vi "StellarNet sw.ini Params.vi"(8 "Error State (In)":errorcluster, 11 "configuration file path":path=path "C:/program files/StellarNet/SpectraWiz/sw.ini") -> (0 "Error State (Out)":errorcluster, 1 "Channel Specific Data- Truncation Settings":cluster{"value":i32, "value":i32}[](array[cluster]), 2 "Channel\nParameters":T1(array[cluster]), 3 "Number of Channels":i32=3, 4 "Spectrometer Wavelengths":dbl[][](array[numeric]) format="%.2f", 5 "file or folder exists?":bool, 7 "Coefficients":ext[][](array[numeric]))   [LabVIEW 2023]
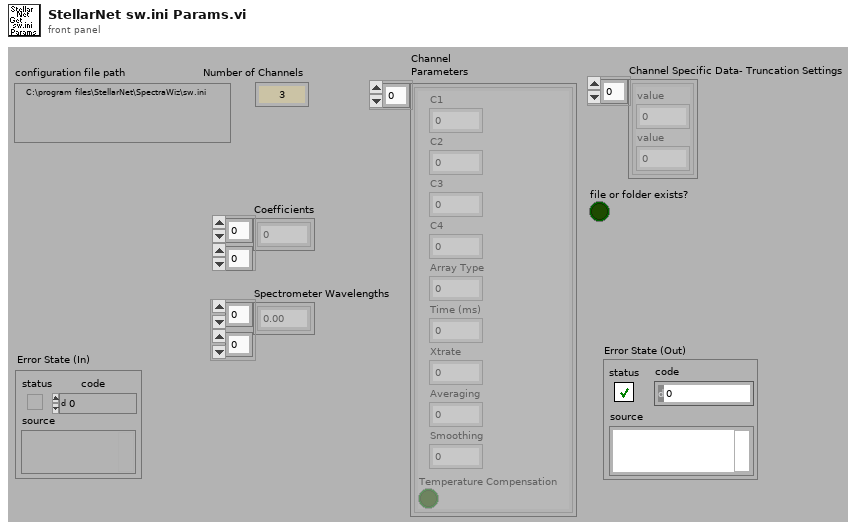
[diagram p1: front panel]
types:
  T1 = cluster{"C1":dbl, "C2":dbl, "C3":dbl, "C4":dbl, "Array Type":u16, "Time (ms)":i32, "Xtrate":i32, "Averaging":i32, "Smoothing":i32, "Temperature Compensation":bool}[]
  T2 = cluster{"C1":dbl, "C2":dbl, "C3":dbl, "C4":dbl, "Array Type":u16, "Time (ms)":i32, "Xtrate":i32, "Averaging":i32, "Smoothing":i32, "Temperature Compensation":bool}
  T3 = cluster{"[0]":dbl, "[1]":dbl, "[2]":dbl, "[3]":dbl, "[4]":dbl, "[5]":dbl, "[6]":dbl, "[7]":dbl, "[8]":dbl}
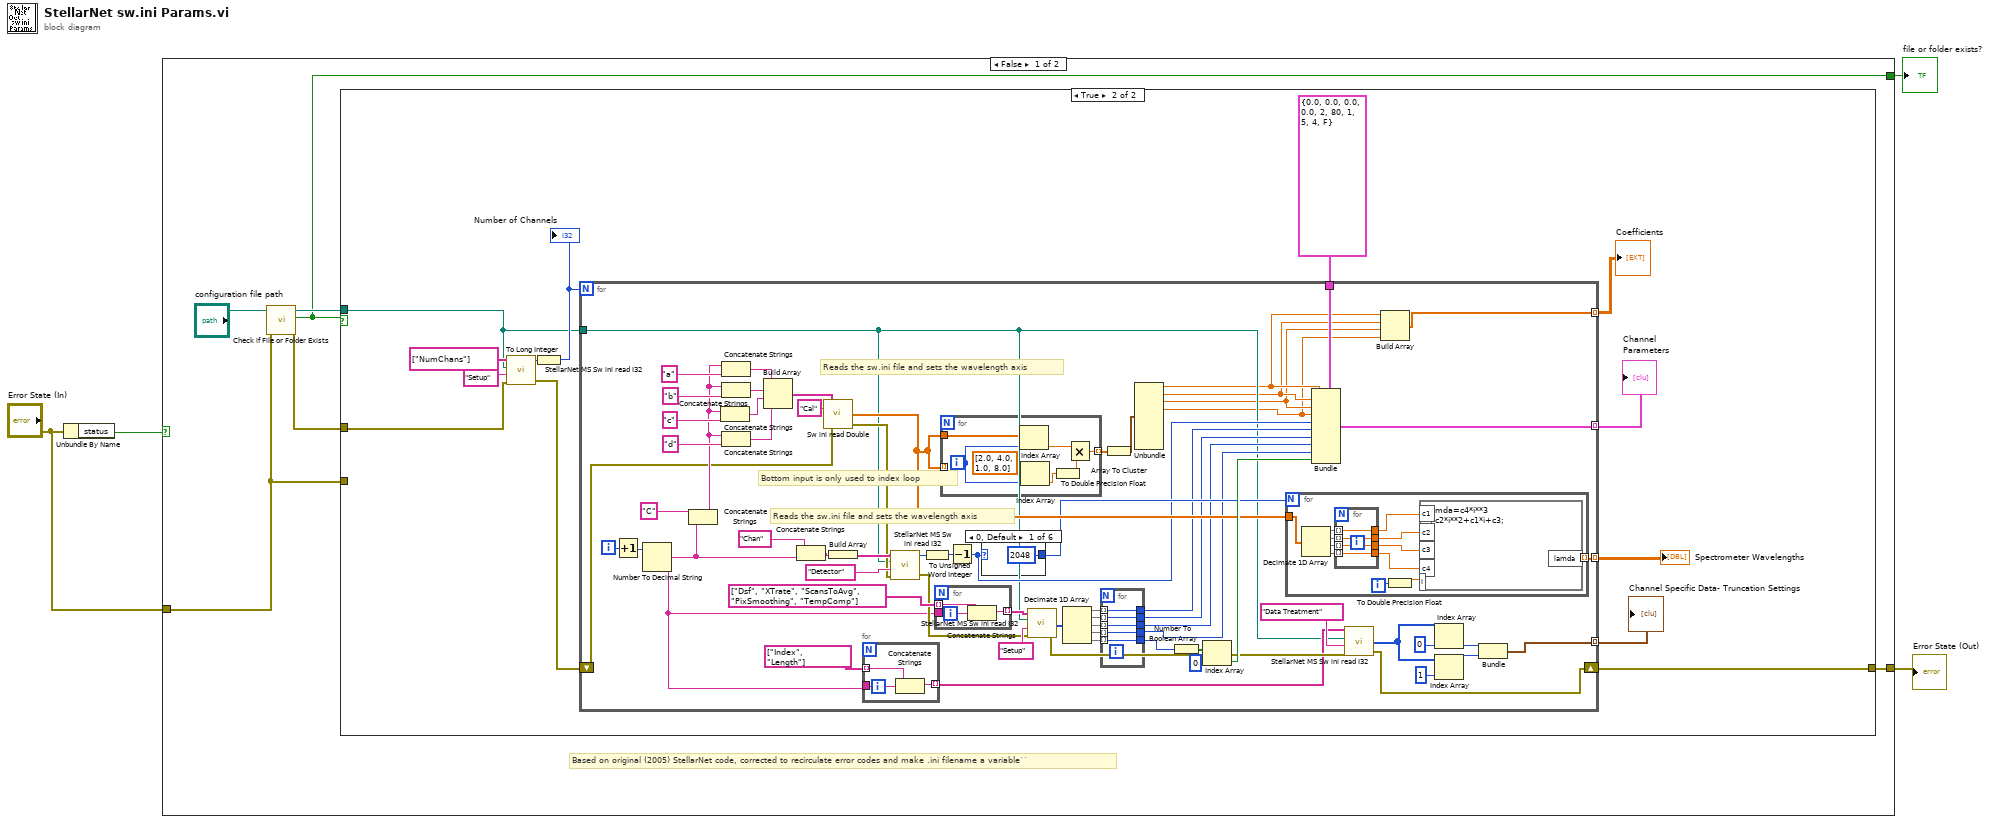
[diagram p0: block diagram]
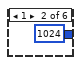
[diagram p3: hidden frame]
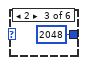
[diagram p4: hidden frame]
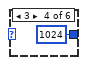
[diagram p5: hidden frame]
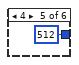
[diagram p6: hidden frame]
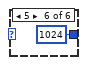
[diagram p7: hidden frame]
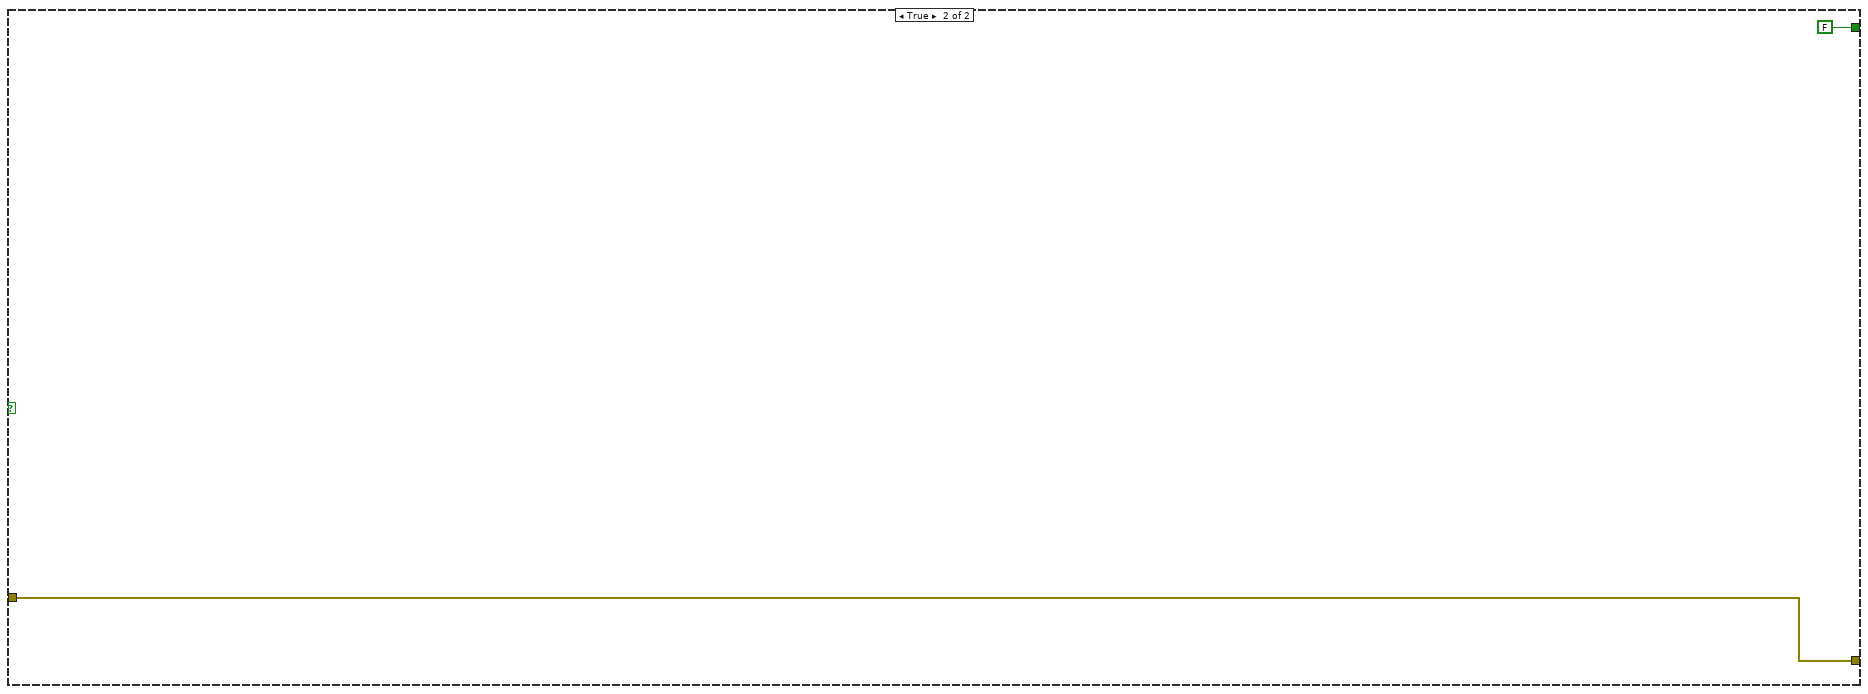
[diagram p8: hidden frame]
diagram:
  n1 = Unbundle By Name("Error State (In)") -> ("status"=w3:bool)
  n2 = case shown="False" w3 {
    tunnel: [w10 w132] -> w4
    tunnel: "Error State (In)" -> [w6 w132]
    tunnel: [w5 FALSE ("file or folder exists?")] -> w1
    frame False {
      # "Based on original (2005) StellarNet code, corrected to recirculate error codes and make .ini filename a variable``"
      n3 = call <vilib>:"Check if File or Folder Exists.vi"("error in (no error)"=w6, "path"="configuration file path") -> ("error out"=w8:errorcluster, "file or folder exists?"=w5:bool, "dup path"=w7:path)  [unwired: 7 in]
      n4 = case shown="True" w5 {
        tunnel: [w11 w19] -> w10
        tunnel: w8 -> [_ w14]
        tunnel: w7 -> [_ w13]
        tunnel: w6 -> [w11 _]
        frame False {
          # "sw.ini not found.  We'll use last-resort defaults and ask the user."
        }
        frame True {
          n5 = call "StellarNet MS Sw ini read I32.vi"("Error State (In)"=w14, "Section"="Setup", "configuration file path"=w13, "Keys"=string[] ["NumChans"]) -> ("Error State (Out)"=w20:errorcluster, "Single Element"=w21:i32)  [unwired: 1 out]
          n6 = To Long Integer(number=w21) -> (32bit integer=w16:i32)
          "Number of Channels" <- w16
          n7 = for {
            N: w16 -> [_]
            tunnel: [w59] -> w17 mode=indexing
            tunnel: [w58] -> w24 mode=indexing
            tunnel: [w34] -> w15 mode=indexing
            shift-right: [w43] -> w19
            shift-left: w20 -> [w51]
            tunnel: T2 {"C1"=0.0, "C2"=0.0, "C3"=0.0, "C4"=0.0, "Array Type"=2, "Time (ms)"=80, "Xtrate"=1, "Averaging"=5, "Smoothing"=4, "Temperature Compensation"=FALSE} ("Cluster") -> [w31]
            tunnel: w13 -> [w30]
            tunnel: [w25] -> w12 mode=indexing
            i -> [w90]
            # "Bottom input is only used to index loop"
            # "Reads the sw.ini file and sets the wavelength axis"
            # "Reads the sw.ini file and sets the wavelength axis"
            n8 = Increment(x=w90) -> (x+1=w89:i32)
            n9 = Number To Decimal String(number=w89) -> (decimal integer string=w40:string)  [unwired: 1 in]
            n10 = Concatenate Strings("C", w40) -> (w83:string)
            n11 = Concatenate Strings(w83, "c") -> (w80:string)
            n12 = Concatenate Strings(w83, "a") -> (w82:string)
            n13 = Concatenate Strings(w83, "b") -> (w81:string)
            n14 = Concatenate Strings(w83, "d") -> (w79:string)
            n15 = Build Array(w82, w81, w80, w79) -> (w63:string[])
            n16 = Concatenate Strings("Chan", w40) -> (w61:string)
            n17 = call "Sw ini read Double.vi"("Error State (In)"=w51, "Section"="Cal", "Keys"=w63) -> ("Error State (Out)"=w53:errorcluster, "Multi Elements"=w57:dbl[])  [unwired: 1 out]
            n18 = Build Array(w61) -> (w62:string[])
            n19 = for {
              tunnel: w40 -> [w93]
              tunnel: [w92] -> w41 mode=indexing
              tunnel: string[] ["Index", "Length"] ("Keys") -> [w91] mode=indexing
              n20 = Concatenate Strings(w91, w93) -> (w92:string)
            }
            n21 = call "StellarNet MS Sw ini read I32.vi"("Error State (In)"=w53, "Section"="Detector", "configuration file path"=w30, "Keys"=w62) -> ("Error State (Out)"=w52:errorcluster, "Single Element"=w65:i32)  [unwired: 1 out]
            n22 = To Unsigned Word Integer(number=w65) -> (unsigned 16bit integer=w33:u16)
            n23 = for {
              tunnel: w40 -> [w125]
              tunnel: [w124] -> w60 mode=indexing
              tunnel: string[] ["Dsf", "XTrate", "ScansToAvg", "PixSmoothing", "TempComp"] ("Keys") -> [w123] mode=indexing
              n24 = Concatenate Strings(w123, w125) -> (w124:string)
            }
            n25 = for {
              tunnel: [w95] -> w56 mode=indexing
              tunnel: w57 -> [w94]
              tunnel: w57 -> [_] mode=indexing
              i -> [w99]
              n26 = Index Array(array=w94, index=w99) -> (element=w98:dbl)
              n27 = Index Array(array=dbl[] [2.0, 4.0, 1.0, 8.0], index=w99) -> (element=w97:dbl)
              n28 = To Double Precision Float(number=w97) -> (double precision float=w96:dbl)
              n29 = Multiply(x=w98, y=w96) -> (x*y=w95:dbl)
            }
            n30 = Decrement(x=w33) -> (x-1=w32:u16)
            n31 = case shown="0, Default" w32 {
              tunnel: [u16 2048 u16 1024 u16 2048 u16 1024 u16 512 u16 1024] -> w54
              frame 0, Default {
              }
              frame 1 {
              }
              frame 2 {
              }
              frame 3 {
              }
              frame 4 {
              }
              frame 5 {
              }
            }
            n32 = call "StellarNet MS Sw ini read I32.vi"("Error State (In)"=w52, "Section"="Setup", "configuration file path"=w30, "Keys"=w60) -> ("Error State (Out)"=w44:errorcluster, "Multi Elements"=w70:i32[])  [unwired: 1 out]
            n33 = Decimate 1D Array(w70) -> (w71:i32[], w72:i32[], w73:i32[], w74:i32[], w75:i32[])
            n34 = for {
              tunnel: [w130] -> w46
              tunnel: w71 -> [w130] mode=indexing
              tunnel: [w129] -> w47
              tunnel: w72 -> [w129] mode=indexing
              tunnel: [w128] -> w48
              tunnel: w73 -> [w128] mode=indexing
              tunnel: [w127] -> w49
              tunnel: w74 -> [w127] mode=indexing
              tunnel: [w126] -> w50
              tunnel: w75 -> [w126] mode=indexing
            }
            n35 = Array To Cluster(array=w56) -> (cluster=w55:T3)
            n36 = Unbundle(w55) -> ("[0]"=w29:dbl, "[1]"=w28:dbl, "[2]"=w27:dbl, "[3]"=w26:dbl)  [unwired: 5 out]
            n37 = Number To Boolean Array(number=w50) -> (Boolean array=w76:bool[])
            n38 = Index Array(array=w76, index=0) -> (element=w64:bool)
            n39 = for {
              N: w54 -> [_]
              tunnel: [w110] -> w58 mode=indexing
              tunnel: w57 -> [w109]
              i -> [w112]
              n40 = Decimate 1D Array(w109) -> (w106:dbl[], w107:dbl[], w108:dbl[], w105:dbl[])
              n41 = for {
                tunnel: [w116] -> w102
                tunnel: w108 -> [w116] mode=indexing
                tunnel: w107 -> [w115] mode=indexing
                tunnel: [w115] -> w103
                tunnel: [w114] -> w104
                tunnel: w106 -> [w114] mode=indexing
                tunnel: [w113] -> w101
                tunnel: w105 -> [w113] mode=indexing
              }
              n42 = To Double Precision Float(number=w112) -> (double precision float=w111:dbl)
              n43 = formula code="lamda=c4*i**3\n+c2*i**2+c1*i+c3;"("c2"=w103, "c3"=w102, "c4"=w101, "i"=w111, "c1"=w104) -> ("lamda"=w110:dbl)
            }
            n44 = Bundle(cluster=w31, "C1"=w29, "C2"=w28, "C3"=w27, "C4"=w26, "Array Type"=w32, "Time (ms)"=w46, "Xtrate"=w47, "Averaging"=w48, "Smoothing"=w49, "Temperature Compensation"=w64) -> (w59:T2)
            n45 = call "StellarNet MS Sw ini read I32.vi"("Error State (In)"=w44, "Section"="Data Treatment", "configuration file path"=w30, "Keys"=w41) -> ("Error State (Out)"=w43:errorcluster, "Multi Elements"=w37:i32[])  [unwired: 1 out]
            n46 = Build Array(w29, w28, w27, w26) -> (w25:dbl[])
            n47 = Index Array(array=w37, index=0) -> (element=w35:i32)
            n48 = Index Array(array=w37, index=1) -> (element=w36:i32)
            n49 = Bundle("value"=w35, "value"=w36) -> (w34:cluster{"value":i32, "value":i32})  [unwired: 1 in]
          }
          "Spectrometer Wavelengths" <- w24
          "Channel Specific Data- Truncation Settings" <- w15
          "Channel\nParameters" <- w17
          "Coefficients" <- w12
        }
      }
    }
    frame True {
    }
  }
  "Error State (Out)" <- w4
  "file or folder exists?" <- w1
